vi "showGrid.vi"(6 "Append Text? (True)":bool, 7 "Color (Red)":u32(colorbox), 8 "error in (no error)":errorcluster, 9 "Rows (Default: 3)":i32=3, 10 "Cols (Default: 2)":i32=2, 11 "Image":T2) -> (0 "error out":errorcluster, 3 "Original":T2(plugin-control), 5 "ROIs":T1(array[cluster]))   [LabVIEW 2018]
uses:
  <vilib>/vision/Image Controls.llb/IMAQ Image.ctl
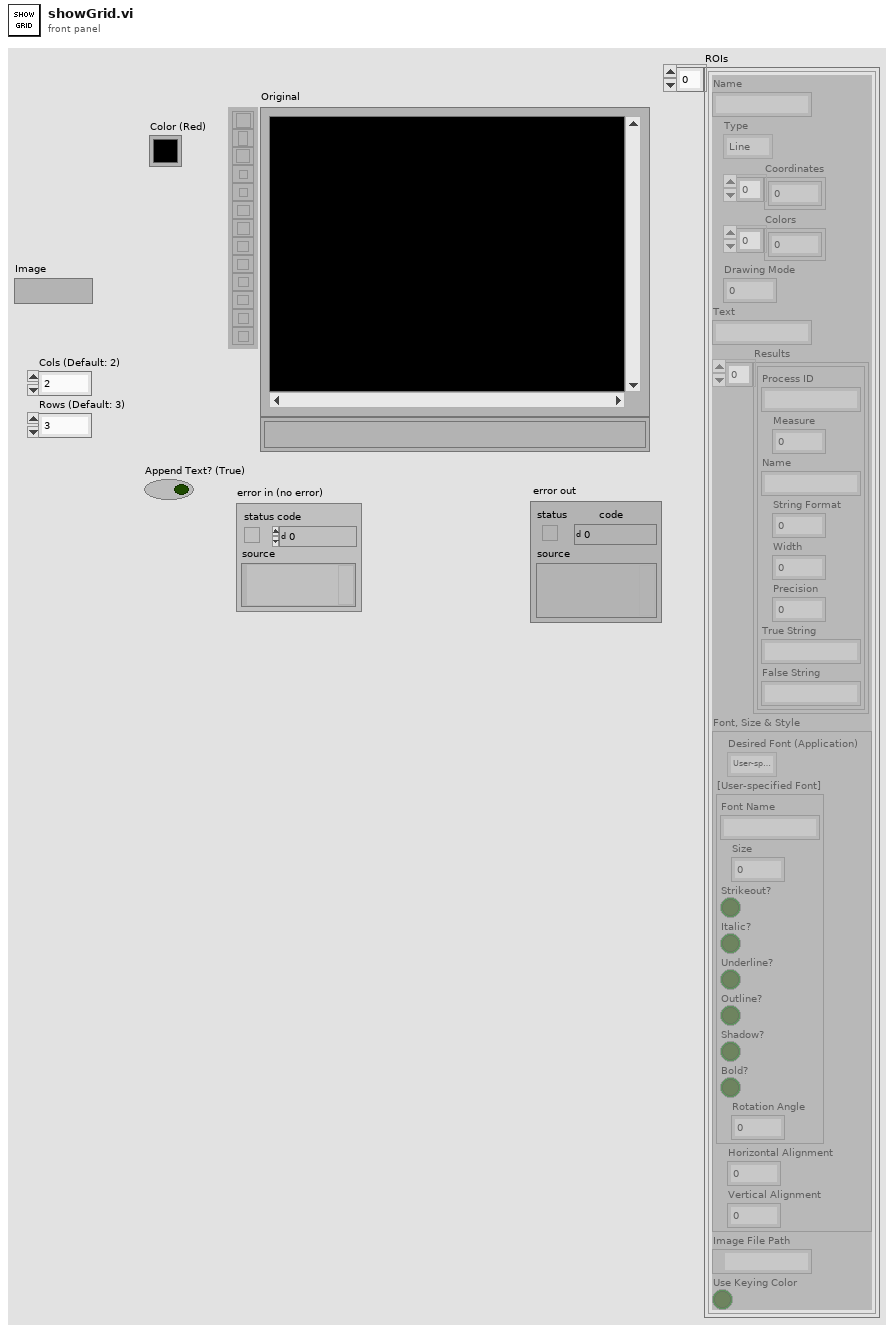
[diagram p1: front panel]
types:
  T1 = cluster{"Name":string, "Type":enum16{"Line", "Broken Line", "Free Hand Line", "Rotated Rectangle", "Oval", "Polygon", "Free Hand", "Bitmap", "Text"}, "Coordinates":i32[], "Colors":u32[], "Drawing Mode":u32, "Text":string, "Results":cluster{"Process ID":string, "Measure":u16, "Name":string, "String Format":u16, "Width":i16, "Precision":i16, "True String":string, "False String":string}[], "Font, Size & Style":cluster{"Desired Font (Application)":enum16{"User-specified Font", "Application Font", "System Font", "Dialog Font"}, "[User-specified Font]":cluster{"Font Name":string, "Size":i16, "Strikeout?":bool, "Italic?":bool, "Underline?":bool, "Outline?":bool, "Shadow?":bool, "Bold?":bool, "Rotation Angle":dbl}, "Horizontal Alignment":i16, "Vertical Alignment":i16}, "Image File Path":path, "Use Keying Color":bool}[]
  T2 = typedef "IMAQ Image.ctl" = refnum<image>
  T3 = cluster{"Name":string, "Type":enum16{"Line", "Broken Line", "Free Hand Line", "Rotated Rectangle", "Oval", "Polygon", "Free Hand", "Bitmap", "Text"}, "Coordinates":i32[], "Colors":u32[], "Drawing Mode":u32, "Text":string, "Results":cluster{"Process ID":string, "Measure":u16, "Name":string, "String Format":u16, "Width":i16, "Precision":i16, "True String":string, "False String":string}[], "Font, Size & Style":cluster{"Desired Font (Application)":enum16{"User-specified Font", "Application Font", "System Font", "Dialog Font"}, "[User-specified Font]":cluster{"Font Name":string, "Size":i16, "Strikeout?":bool, "Italic?":bool, "Underline?":bool, "Outline?":bool, "Shadow?":bool, "Bold?":bool, "Rotation Angle":dbl}, "Horizontal Alignment":i16, "Vertical Alignment":i16}, "Image File Path":path, "Use Keying Color":bool}
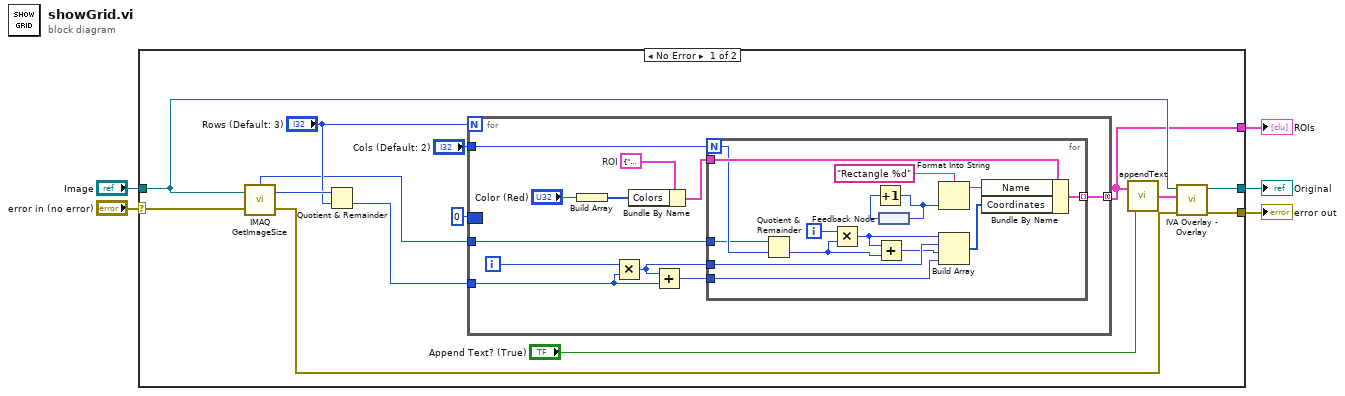
[diagram p0: block diagram]
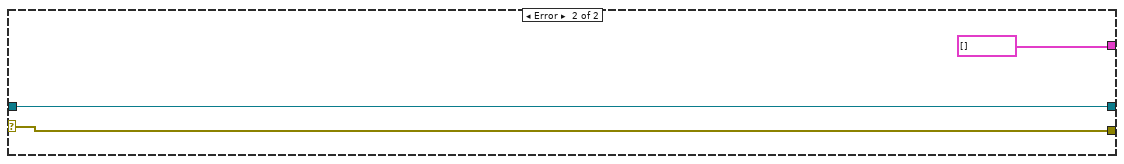
[diagram p2: hidden frame]
diagram:
  n1 = case shown="No Error" "error in (no error)" {
    selector: "error in (no error)" -> [w9 w48]
    tunnel: [w17 w47] -> w5
    tunnel: "Image" -> [w11 w47]
    tunnel: [w8 w48] -> w2
    tunnel: [w7 T1 []] -> w1
    frame No Error {
      n2 = call "IMAQ GetImageSize"("Image"=w11, "error in (no error)"=w9) -> ("Y Resolution"=w19:i32, "X Resolution"=w15:i32, "error out"=w10:errorcluster)  [unwired: 2 in]
      n3 = Quotient & Remainder(x=w19, y="Rows (Default: 3)") -> (floor(x/y)=w18:i32)  [unwired: 1 out]
      n4 = for {
        N: "Rows (Default: 3)" -> [_]
        tunnel: w18 -> [w30]
        tunnel: [w27] -> w7 mode=concatenating
        tunnel: w15 -> [w25]
        border: 0 -> [_]
        tunnel: "Cols (Default: 2)" -> [w24]
        i -> [w26]
        w21 = T3 {"Name"="", "Type"=enum."Rotated Rectangle", "Coordinates"=[], "Colors"=[16711680], "Drawing Mode"=0, "Text"="fgfgf", "Results"=[], "Font, Size & Style"={"Desired Font (Application)"=enum."System Font", "[User-specified Font]"={"Font Name"="Tahoma", "Size"=13, "Strikeout?"=FALSE, "Italic?"=FALSE, "Underline?"=FALSE, "Outline?"=FALSE, "Shadow?"=FALSE, "Bold?"=FALSE, "Rotation Angle"=0.0}, "Horizontal Alignment"=0, "Vertical Alignment"=0}, "Image File Path"=path "", "Use Keying Color"=FALSE}  # ROI
        n5 = Build Array("Color (Red)") -> (w22:u32[])
        n6 = Multiply(x=w26, y=w30) -> (x*y=w28:i32)
        n7 = Bundle By Name(cluster=w21, "Colors"=w22) -> (w20:T3)
        n8 = Add(x=w28, y=w30) -> (x+y=w29:i32)
        n9 = for {
          N: w24 -> [w34]
          tunnel: w20 -> [w45]
          tunnel: w29 -> [w38]
          tunnel: w28 -> [w40]
          tunnel: [w36] -> w27 mode=indexing
          tunnel: w25 -> [w33]
          i -> [w42]
          n10 = Quotient & Remainder(x=w33, y=w34) -> (floor(x/y)=w35:i32)  [unwired: 1 out]
          n11 = Multiply(x=w42, y=w35) -> (x*y=w41:i32)
          n12 = Add(x=w41, y=w35) -> (x+y=w39:i32)
          n13 = feedback #1() -> (w31:i32)
          n14 = Increment(x=w31) -> (x+1=w32:i32)
          n15 = feedback-in #1(w32) -> ()
          n16 = Format Into String(format string="Rectangle %d", w32) -> (resulting string=w43:string)  [unwired: 2 in, 1 out]
          n17 = Build Array(w41, w40, w39, w38) -> (w37:i32[])
          n18 = Bundle By Name(cluster=w45, "Name"=w43, "Coordinates"=w37) -> (w36:T3)
        }
      }
      n19 = call "appendText.vi"("Append?"="Append Text? (True)", "Array in"=w7) -> ("Array out"=w12:T1)
      n20 = call <vilib>:"IVA Overlay - Overlay.vi"("error in (no error)"=w10, "Parameters"=w12, "Image In"=w11) -> ("error out"=w8:errorcluster, "Image Out"=w17:T2)  [unwired: 7 out]
    }
    frame Error {
    }
  }
  "Original" <- w5
  "error out" <- w2
  "ROIs" <- w1
